vi "Service Values.vi"(11 "Service in":refnum<class "Service.lvclass">) -> (2 "ID":string, 3 "Type":string)   [LabVIEW 2020, in "Vecto.lvlib" / "Service.lvclass"]
uses:
  Service.lvclass
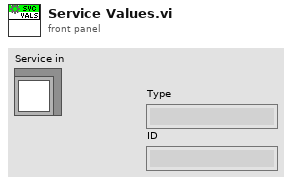
[diagram p1: front panel]
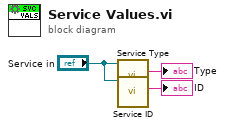
[diagram p0: block diagram]
diagram:
  n1 = call-dynamic "Service Type.vi"("Service in"="Service in") -> ("Type"=→"Type":string)  [unwired: 10 in]
  n2 = call-dynamic "Service ID.vi"("Service in"="Service in") -> ("ID"=→"ID":string)  [unwired: 10 in]
